vi "Header or Footer.vi"(0 "OverContent":refnum<k24>, 2 "Header or Footer":T1, 5 "NumberOfPages":i32=1, 7 "pageNum":i32=1, 9 "Header or Footer Complete Cluster":T2, 11 "error in (no error)":errorcluster) -> (4 "OverContent duplicate":refnum<k24>, 15 "error out":errorcluster)   [LabVIEW 2012]
doc: "Version 1.0\nDeveloped by Jean-Marc Simard\nCopyright © 2010, Exaprom Inc.\nAll rights reserved.\nLicense: BSD\n\nWith iTextSharp 4.1.6 (http://itextsharp.sourceforge.net)\nunder Mozilla Public License Version 1.1\n(http://www.mozilla.org/MPL/MPL-1.1.html)"
uses:
  C:/Users/MaxCorp/Documents/TopPerm - Base/DLL/itextsharp.dll
  DLL/itextsharp.dll
  Controls/Header Footer Complete Cluster.ctl
  Controls/Header Footer Cluster with references.ctl
  Controls/Header Footer Type.ctl
  Controls/Header footer horiz alignment.ctl
  Controls/Cell Vertical alignment.ctl
  Controls/Page number.ctl
  Controls/Font cluster.ctl
  Controls/Font size.ctl
  Controls/Font color.ctl
  Controls/Header Footer Line.ctl
  Controls/Header or Footer.ctl
panel:
  # "X"
  # "Y"
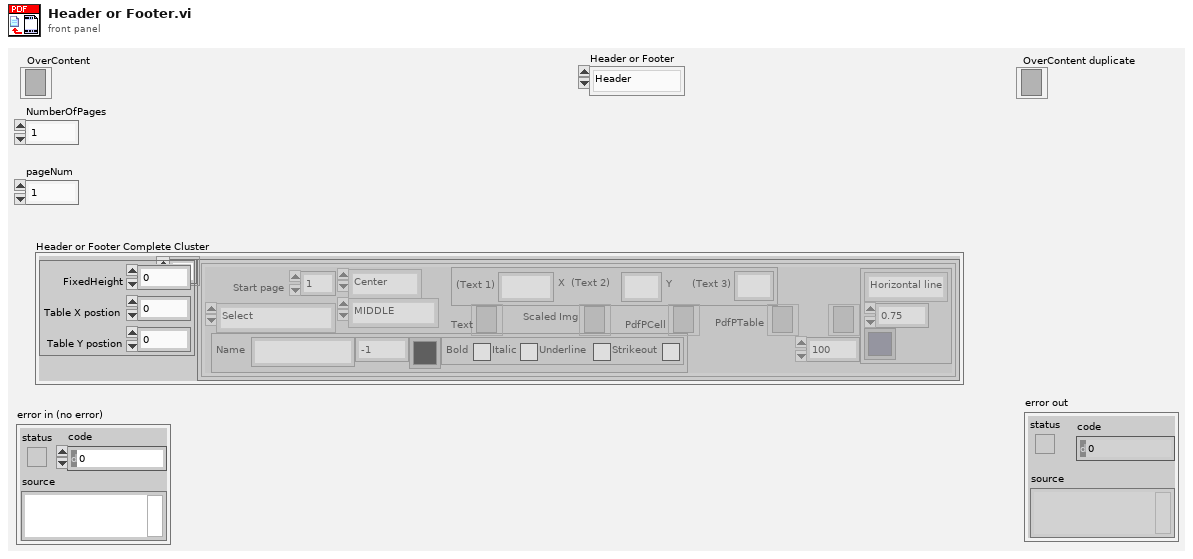
[diagram p1: front panel]
types:
  T1 = typedef "Header or Footer.ctl" = enum16{"Header", "Footer"}
  T2 = typedef "Header Footer Complete Cluster.ctl" = cluster{"Table position":cluster{"FixedHeight":dbl, "Table X postion":dbl, "Table Y postion":dbl}, "Header Footer Cluster with references [ ]":T3[]}
  T3 = typedef "Header Footer Cluster with references.ctl" = cluster{"Start page":i32, "Type":T4, "Alignment":T5, "Vertical Alignement":T6, "Page #":T7, "Text":refnum<k24>, "Scaled Img":refnum<k24>, "PdfPCell":refnum<k24>, "PdfPTable":refnum<k24>, "Font Cluster":T8, "Font ":refnum<k24>, "Img (%)":sgl, "Line":cluster{"Line":T11, "Thickness (points)":sgl, "Colour":T10}}
  T4 = typedef "Header Footer Type.ctl" = enum16{"Select", "Text", "Text + hyperlink", "Page number", "Image", "Image + hyperlink"}
  T5 = typedef "Header footer horiz alignment.ctl" = enum16{"Left", "Center", "Right"}
  T6 = typedef "Cell Vertical alignment.ctl" = enum16{"TOP", "MIDDLE", "BOTTOM"}
  T7 = typedef "Page number.ctl" = cluster{"Text 1":string, "Text 2":string, "Text 3":string}
  T8 = typedef "Font cluster.ctl" = cluster{"Name":string, "Size":T9, "Color":T10, "Style":cluster{"Bold":bool, "Italic":bool, "Underline":bool, "Strikeout":bool}}
  T9 = typedef "Font size.ctl" = sgl
  T10 = typedef "Font color.ctl" = u32
  T11 = typedef "Header Footer Line.ctl" = enum16{"No line", "Horizontal line"}
  T12 = cluster{"FixedHeight":dbl, "Table X postion":dbl, "Table Y postion":dbl}
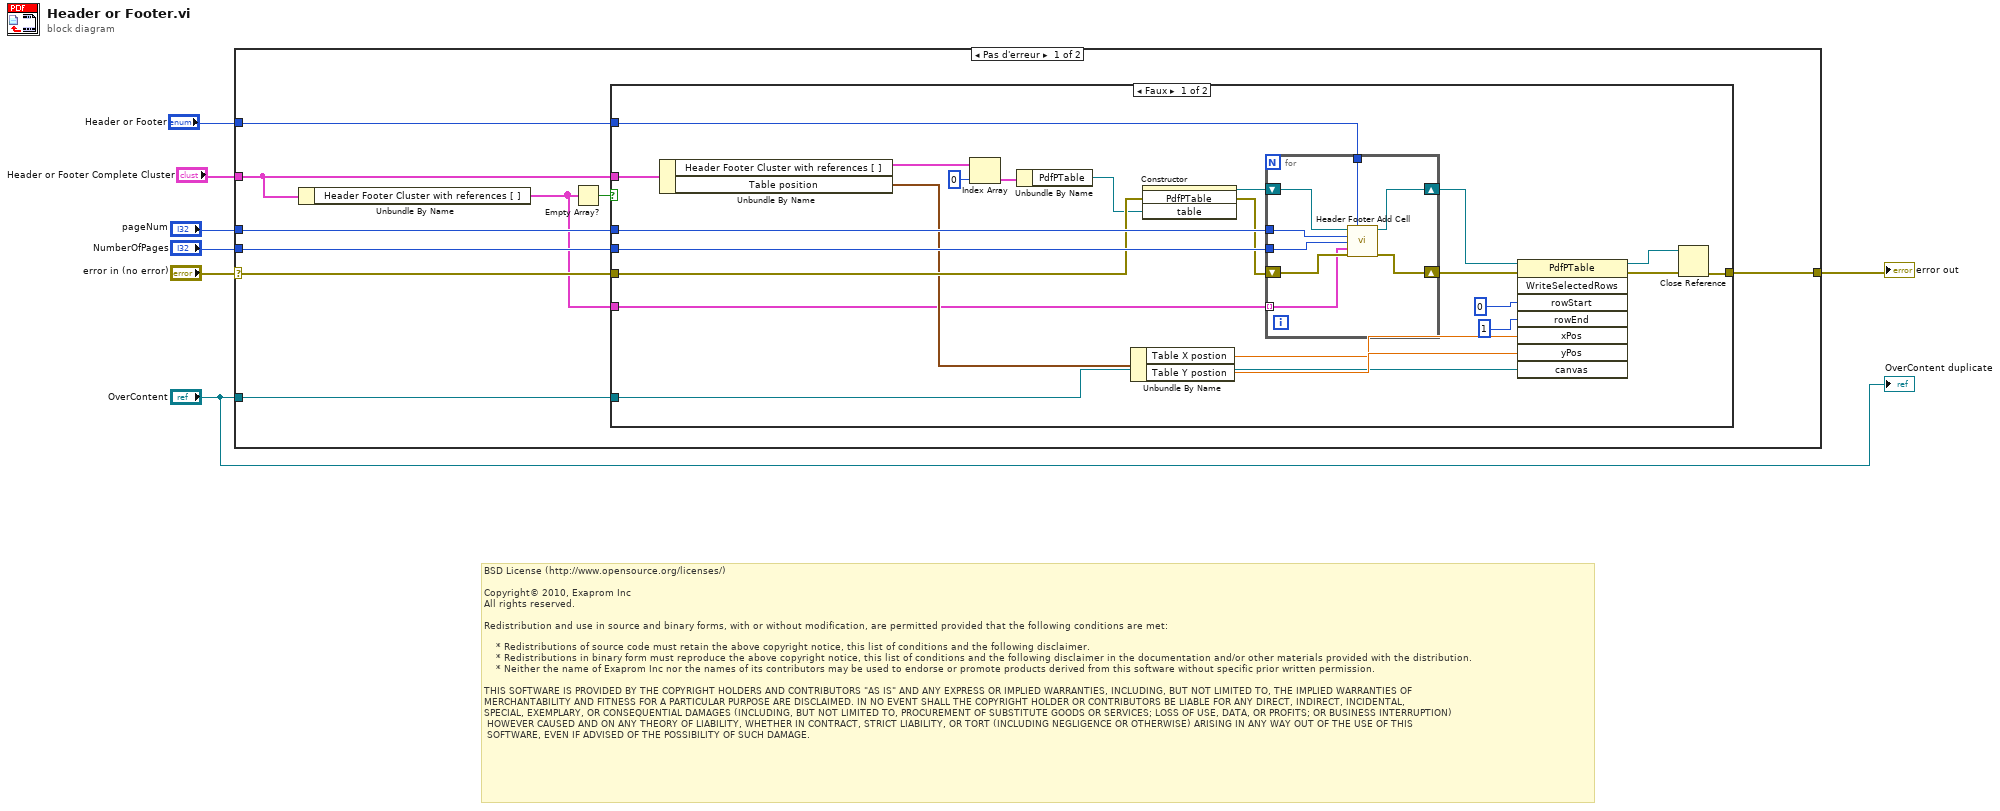
[diagram p0: block diagram]
diagram:
  # "BSD License (http://www.opensource.org/licenses/)\n\nCopyright© 2010, Exaprom Inc\nAll rights reserved.\n\nRedistribution and use in source and binary forms, with or without modification, are permitted provided that the following conditions are met:\n\n    * Redistributions of source code must retain the above copyright notice, this list of conditions and the following disclaimer.\n    * Redistributions in binary form must reproduce the above copyright notice, this list of conditions and the following disclaimer in the documentation and/or other materials provided with the distribution.\n    * Neither the name of Exaprom Inc nor the names of its contributors may be used to endorse or promote products derived from this software without specific prior written permission.\n\nTHIS SOFTWARE IS PROVIDED BY THE COPYRIGHT HOLDERS AND CONTRIBUTORS \"AS IS\" AND ANY EXPRESS OR IMPLIED WARRANTIES, INCLUDING, BUT NOT LIMITED TO, THE IMPLIED WARRANTIES OF \nMERCHANTABILITY AND FITNESS FOR A PARTICULAR PURPOSE ARE DISCLAIMED. IN NO EVENT SHALL THE COPYRIGHT HOLDER OR CONTRIBUTORS BE LIABLE FOR ANY DIRECT, INDIRECT, INCIDENTAL,\nSPECIAL, EXEMPLARY, OR CONSEQUENTIAL DAMAGES (INCLUDING, BUT NOT LIMITED TO, PROCUREMENT OF SUBSTITUTE GOODS OR SERVICES; LOSS OF USE, DATA, OR PROFITS; OR BUSINESS INTERRUPTION)\n HOWEVER CAUSED AND ON ANY THEORY OF LIABILITY, WHETHER IN CONTRACT, STRICT LIABILITY, OR TORT (INCLUDING NEGLIGENCE OR OTHERWISE) ARISING IN ANY WAY OUT OF THE USE OF THIS\n SOFTWARE, EVEN IF ADVISED OF THE POSSIBILITY OF SUCH DAMAGE."
  n1 = case shown="Pas d'erreur" "error in (no error)" {
    selector: "error in (no error)" -> [w14 w49]
    tunnel: [w15 w49] -> w7
    tunnel: "pageNum" -> [w16 _]
    tunnel: "OverContent" -> [w13 _]
    tunnel: "NumberOfPages" -> [w12 _]
    tunnel: "Header or Footer Complete Cluster" -> [w11 _]
    tunnel: "Header or Footer" -> [w10 _]
    frame No Error {
      n2 = Unbundle By Name(w11) -> ("Header Footer Cluster with references [ ]"=w8:T3[])
      n3 = Empty Array?(array=w8) -> (empty?=w9:bool)
      n4 = case shown="Faux" w9 {
        tunnel: w16 -> [w36 _]
        tunnel: [w26 w48] -> w15
        tunnel: w14 -> [w31 w48]
        tunnel: w13 -> [w33 _]
        tunnel: w12 -> [w32 _]
        tunnel: w11 -> [w25 _]
        tunnel: w8 -> [w23 _]
        tunnel: w10 -> [w21 _]
        frame False {
          n5 = Unbundle By Name(w25) -> ("Header Footer Cluster with references [ ]"=w20:T3[], "Table position"=w24:T12)
          n6 = Index Array(array=w20, index=0) -> (element=w18:T3)
          n7 = Unbundle By Name(w18) -> ("PdfPTable"=w17:refnum<k24>)
          n8 = Unbundle By Name(w24) -> ("Table X postion"=w34:dbl, "Table Y postion"=w35:dbl)
          n9 = constructor class="PdfPTable"(error in=w31, "table"=w17) -> (reference out=w29:refnum<k24>, error out=w30:errorcluster)  [unwired: 2 in, 2 out]
          n10 = for {
            shift-right: [w44] -> w22
            shift-left: w29 -> [w45]
            shift-right: [w43] -> w37
            shift-left: w30 -> [w47]
            tunnel: w23 -> [w41] mode=indexing
            tunnel: w36 -> [w46]
            tunnel: w32 -> [w42]
            tunnel: w21 -> [w40]
            n11 = call "Header Footer Add Cell.vi"("PdfP Table"=w45, "Header or Footer"=w40, "Page #"=w46, "Total page #"=w42, "Header Footer Cluster with references"=w41, "error in (no error)"=w47) -> ("PdfP Table duplicate"=w44:refnum<k24>, "error out"=w43:errorcluster)  [unwired: 4 in, 4 out]
          }
          n12 = invoke class="PdfPTable" method="WriteSelectedRows"(reference=w22, error in=w37, "rowStart"=0, "rowEnd"=1, "xPos"=w34, "yPos"=w35, "canvas"=w33) -> (reference out=w27:refnum<k24>, error out=w28:errorcluster)  [unwired: 1 in, 6 out]
          n13 = Close Reference(reference=w27, error in (no error)=w28) -> (error out=w26:errorcluster)
        }
        frame True {
        }
      }
    }
    frame Error {
    }
  }
  "error out" <- w7
  "OverContent duplicate" <- "OverContent"
